vi "Measure.vi"(8 "error in":errorcluster, 11 "VISA Interface in":refnum<class "VISA Interface.lvclass">) -> (0 "error out":errorcluster, 2 "Measurement Results":T1={"Voltage (V)"=1.0} {"Voltage (V)" min=-424.2 max=424.2 step=1.0 format="%#.1f"}, 3 "VISA Interface out":refnum<class "VISA Interface.lvclass">)   [LabVIEW 2020, in "Plugin Instrument Driver.lvlib" / "VISA Interface.lvclass"]
doc: "Read Input channel."
uses:
  VISA Interface.lvclass
  C:/SVN_LabSys/labsys_lvcode/LabSys_SourceCode/Plugin Template/Source/Drivers/Instrument Driver/Instrument Driver.lvclass
  Typedefs/Measurement Results.ctl
  Instrument Driver.lvclass
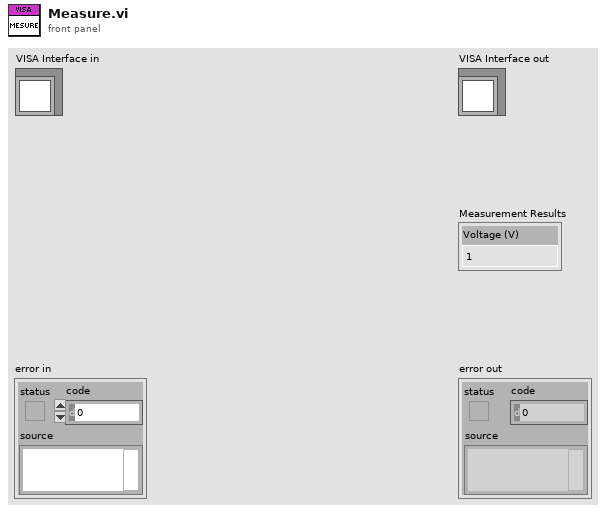
[diagram p1: front panel]
types:
  T1 = typedef "Plugin Instrument Driver.lvlib/Instrument Driver.lvclass/Measurement Results.ctl" = cluster{"Voltage (V)":dbl}
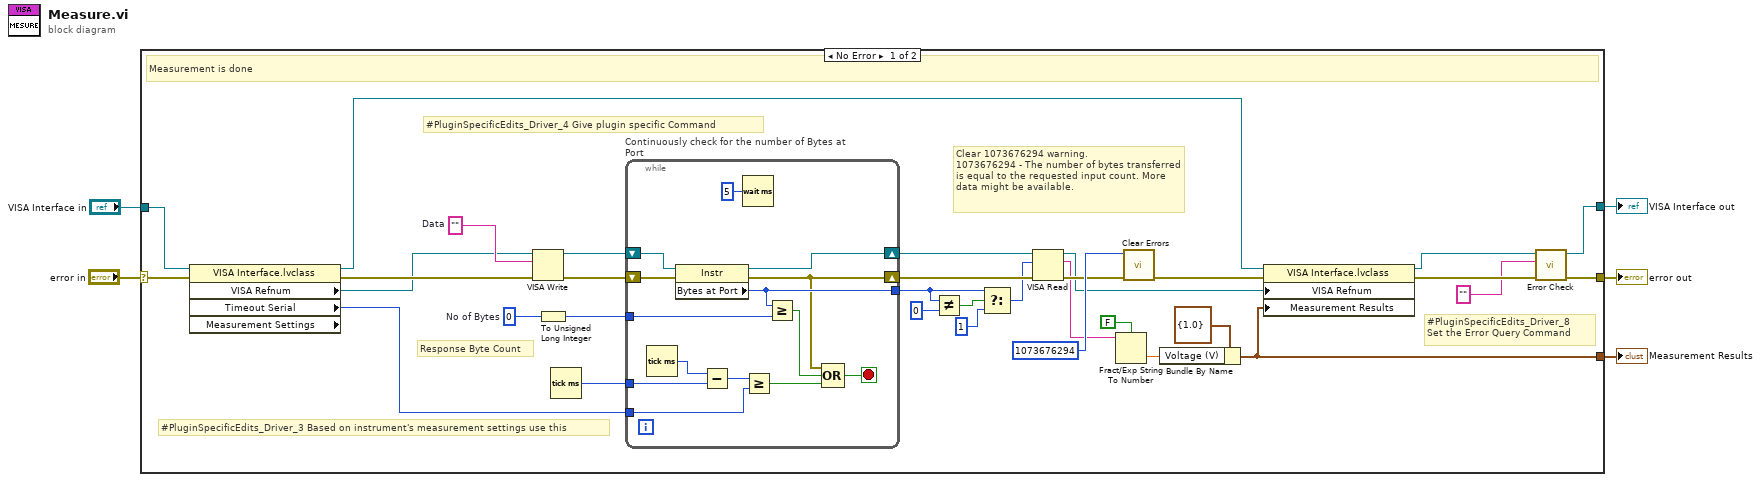
[diagram p0: block diagram]
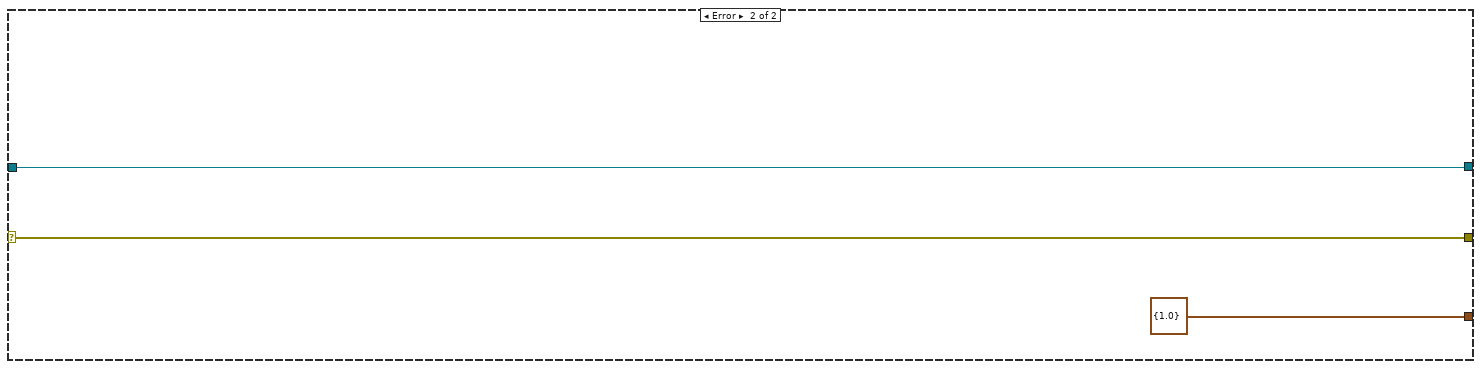
[diagram p2: hidden frame]
diagram:
  n1 = case shown="No Error" "error in" {
    selector: "error in" -> [w24 w54]
    tunnel: "VISA Interface in" -> [w25 w55]
    tunnel: [w8 w54] -> w3
    tunnel: [w10 w55] -> w2
    tunnel: [w12 T1 {"Voltage (V)"=1.0} ("Measurement Results")] -> w1
    frame No Error {
      w26 = u32 0  # No of Bytes
      w27 = ""  # Data
      # "#PluginSpecificEdits_Driver_3 Based on instrument's measurement settings use this"
      # "#PluginSpecificEdits_Driver_8 \nSet the Error Query Command"
      # "#PluginSpecificEdits_Driver_4 Give plugin specific Command"
      # "Clear 1073676294 warning.\n1073676294 - The number of bytes transferred is equal to the requested input count. More data might be available."
      # "Response Byte Count"
      # "Measurement is done"
      n2 = property class="VISA Interface.lvclass" props=["VISA Refnum", "Timeout Serial", "Measurement Settings"](reference=w25, error in=w24) -> (reference out=w18:refnum<class "VISA Interface.lvclass">, error out=w23:errorcluster, "VISA Refnum"=w22:refnum<visa-resource-name>, "Timeout Serial"=w21:u32)  [unwired: 1 out]
      n3 = VISA Write(VISA resource name=w22, write buffer=w27, error in (no error)=w23) -> (VISA resource name out=w36:refnum<visa-resource-name>, error out=w38:errorcluster)  [unwired: 1 out]
      n4 = To Unsigned Long Integer(number=w26) -> (unsigned 32bit integer=w33:u32)
      n5 = Tick Count (ms)() -> (millisecond timer value=w34:u32)
      n6 = while "Continuously check for the number of Bytes at Port" {
        tunnel: [w49] -> w28
        shift-right: [w44] -> w37
        shift-left: w38 -> [w52]
        shift-right: [w50] -> w35
        shift-left: w36 -> [w51]
        tunnel: w34 -> [w46]
        tunnel: w33 -> [w40]
        tunnel: w21 -> [w39]
        stop <- w41 stop-if-true
        n7 = Tick Count (ms)() -> (millisecond timer value=w47:u32)
        n8 = property class="Instr"(reference=w51, error in=w52) -> (reference out=w50:refnum<visa-resource-name>, error out=w44:errorcluster, "Bytes at Port"=w49:u32)
        n9 = Subtract(x=w47, y=w46) -> (x-y=w45:u32)
        n10 = Wait (ms)(milliseconds to wait=u32 5) -> ()  [unwired: 1 out]
        n11 = Greater Or Equal?(x=w45, y=w39) -> (x >= y?=w42:bool)
        n12 = Greater Or Equal?(x=w49, y=w40) -> (x >= y?=w43:bool)
        n13 = Compound Arithmetic op=OR(w44, w43, w42) -> (w41:bool)
      }
      n14 = Not Equal?(x=w28, y=u32 0) -> (x != y?=w31:bool)
      n15 = Select(t=w28, s=w31, f=u32 1 ("t")) -> (s? t:f=w30:u32)
      n16 = VISA Read(VISA resource name=w35, byte count=w30, error in (no error)=w37) -> (VISA resource name out=w16:refnum<visa-resource-name>, read buffer=w15:string, error out=w19:errorcluster)  [unwired: 1 out]
      n17 = Fract/Exp String To Number(use system decimal point (T)=FALSE, string=w15) -> (number=w13:dbl)  [unwired: 2 in, 1 out]
      n18 = call <vilib>:"Clear Errors.vi"("error in (no error)"=w19, "specific error code to clear (0: all)"=1073676294) -> ("error out"=w17:errorcluster)  [unwired: 4 in, 1 out]
      n19 = Bundle By Name(cluster=T1 {"Voltage (V)"=1.0} ("Measurement Results"), "Voltage (V)"=w13) -> (w12:T1)
      n20 = property class="VISA Interface.lvclass"(reference=w18, error in=w17, "VISA Refnum"=w16, "Measurement Results"=w12) -> (reference out=w11:refnum<class "VISA Interface.lvclass">, error out=w9:errorcluster)
      n21 = call "Error Check.vi"("error in"=w9, "Error Query Command"="", "VISA Interface in"=w11) -> ("error out"=w8:errorcluster, "VISA Interface out"=w10:refnum<class "VISA Interface.lvclass">)  [unwired: 7 in]
    }
    frame Error {
    }
  }
  "error out" <- w3
  "VISA Interface out" <- w2
  "Measurement Results" <- w1
